vi "GC EX Vacuum - Step 1.vi"(7 "Step":i32, 8 "error in":errorcluster, 9 "Test Results In":T8, 10 "Gas":T1, 11 "GC Configuration":T2) -> (0 "error out":errorcluster, 1 "Test Results Out":T8, 2 "Gas Out":T1 caption="Gas", 3 "GC Configuration Out":T2)   [LabVIEW 2015]
uses:
  Controls/Test Information.ctl
  Controls/Vacuum Test.ctl
  Controls/Test Timing.ctl
  Controls/Vaccum Thresholds.ctl
  Controls/Helium Test.ctl
  Controls/Helium Thresholds.ctl
  CAN Communication/Gas/Typedefs/Session Handle.ctl
  CAN Communication/Gas/Gas.lvclass
  Controls/Test Results.ctl
  Controls/Step Result.ctl
  SubVIs/Timing/Timing.lvlib
panel:
  out "NI-DAQ Pressure":dbl
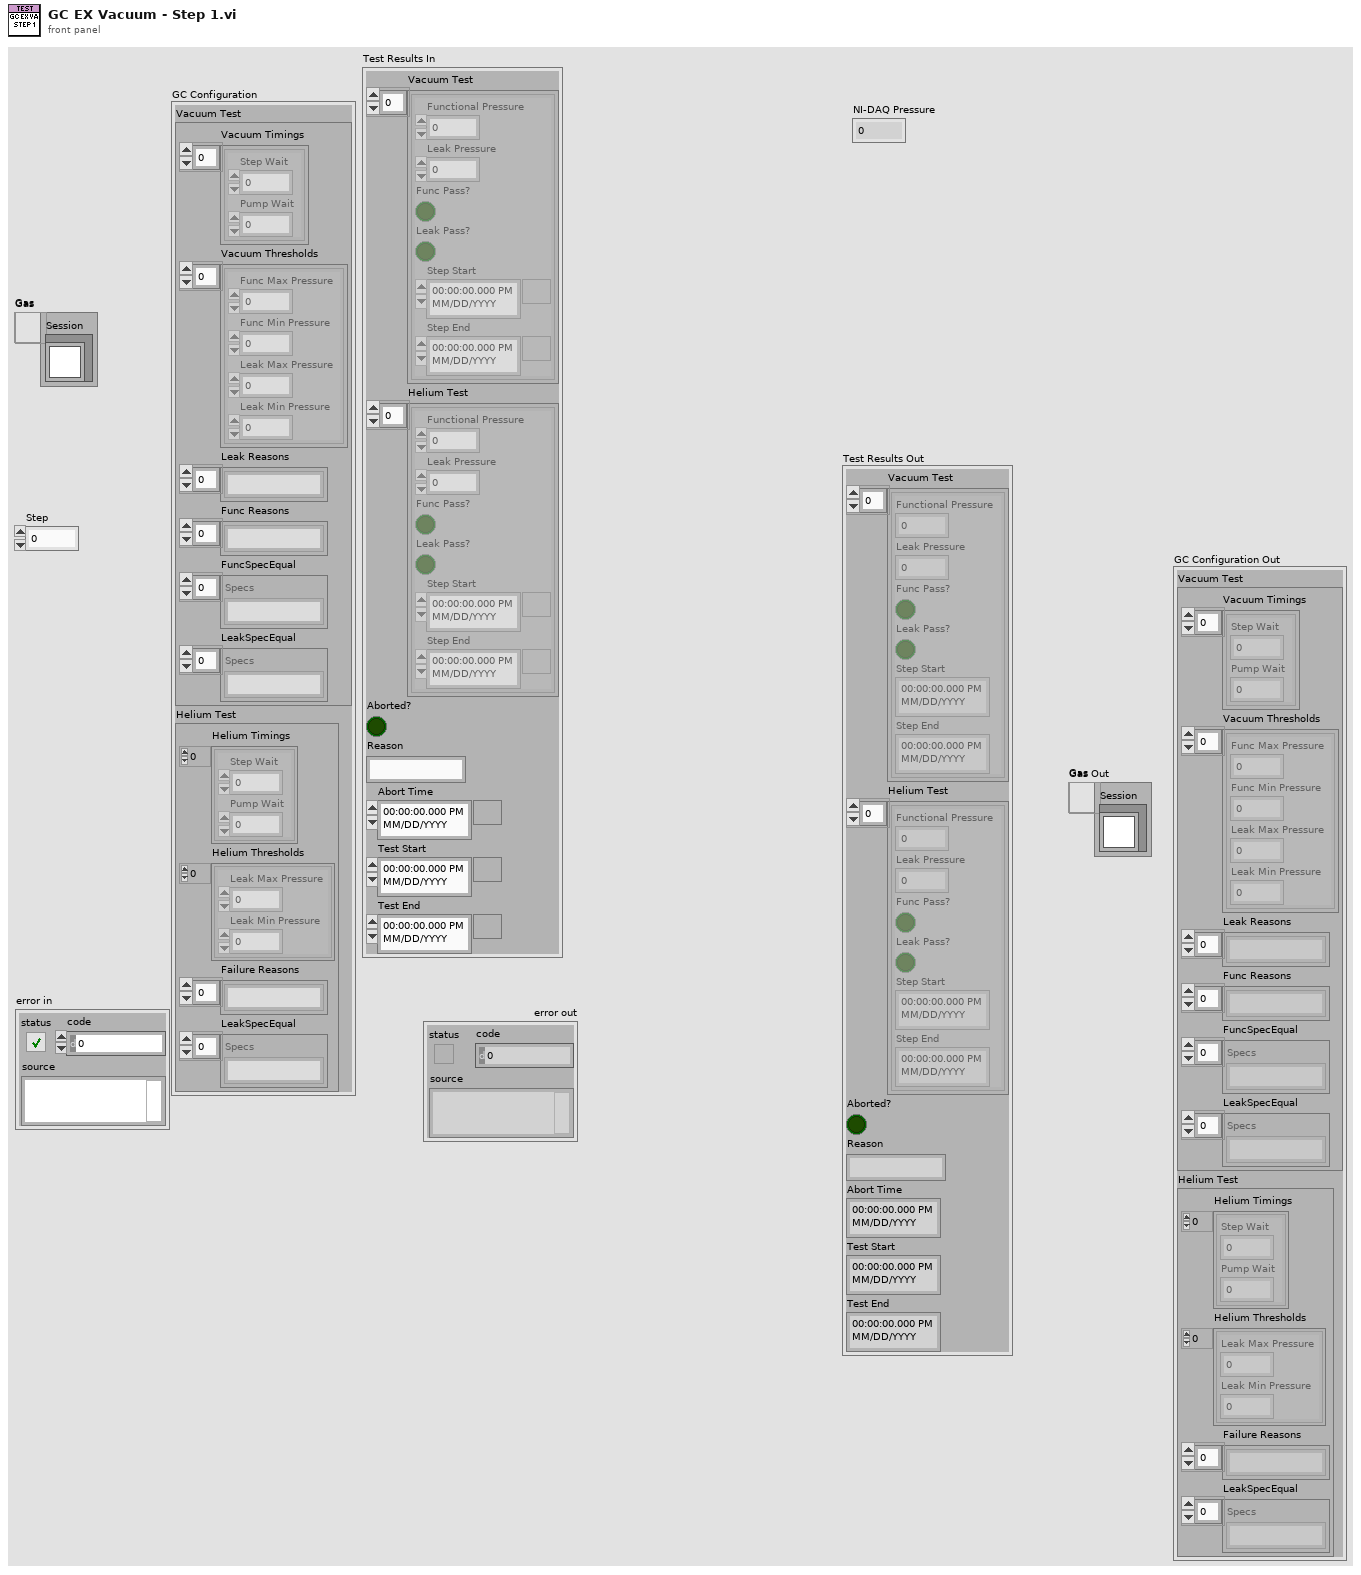
[diagram p1: front panel]
types:
  T1 = typedef "Gas.lvclass/Session Handle.ctl" = refnum<data-value>
  T2 = typedef "Test Information.ctl" = cluster{"Vacuum Test":T3, "Helium Test":T6}
  T3 = typedef "Vacuum Test.ctl" = cluster{"Vacuum Timings":T4[], "Vacuum Thresholds":T5[], "Leak Reasons":string[], "Func Reasons":string[], "FuncSpecEqual":string[], "LeakSpecEqual":string[]}
  T4 = typedef "Test Timing.ctl" = cluster{"Step Wait":dbl, "Pump Wait":dbl}
  T5 = typedef "Vaccum Thresholds.ctl" = cluster{"Func Max Pressure":dbl, "Func Min Pressure":dbl, "Leak Max Pressure":dbl, "Leak Min Pressure":dbl}
  T6 = typedef "Helium Test.ctl" = cluster{"Helium Timings":T4[], "Helium Thresholds":T7[], "Failure Reasons":string[], "LeakSpecEqual":string[]}
  T7 = typedef "Helium Thresholds.ctl" = cluster{"Leak Max Pressure":dbl, "Leak Min Pressure":dbl}
  T8 = typedef "Test Results.ctl" = cluster{"Vacuum Test":T9[], "Helium Test":T9[], "Aborted?":bool, "Reason":string, "Abort Time":timestamp, "Test Start":timestamp, "Test End":timestamp}
  T9 = typedef "Step Result.ctl" = cluster{"Functional Pressure":dbl, "Leak Pressure":dbl, "Func Pass?":bool, "Leak Pass?":bool, "Step Start":timestamp, "Step End":timestamp}
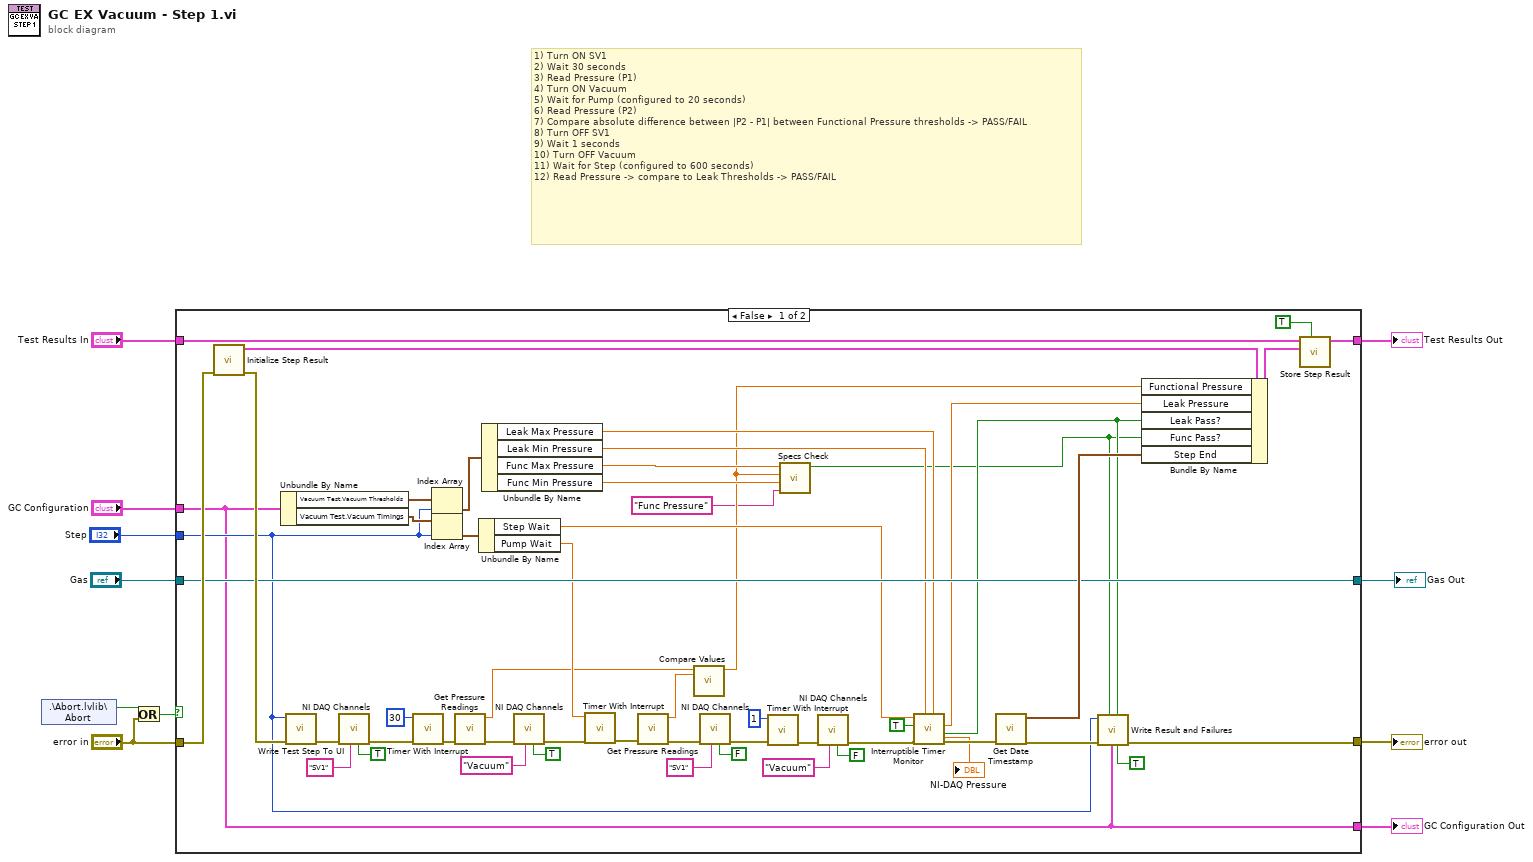
[diagram p0: block diagram]
diagram:
  # "1) Turn ON SV1\n2) Wait 30 seconds\n3) Read Pressure (P1)\n4) Turn ON Vacuum\n5) Wait for Pump (configured to 20 seconds)\n6) Read Pressure (P2)\n7) Compare absolute difference between |P2 - P1| between Functional Pressure thresholds -> PASS/FAIL\n8) Turn OFF SV1\n9) Wait 1 seconds\n10) Turn OFF Vacuum\n11) Wait for Step (configured to 600 seconds)\n12) Read Pressure -> compare to Leak Thresholds -> PASS/FAIL"
  n1 = shared-variable ".\\Abort.lvlib\\Abort"() -> (w10:bool)  [unwired: 1 in, 1 out]
  n2 = Or(x=w10, y="error in") -> (x .or. y?=w9:bool)
  n3 = case shown="False" w9 {
    tunnel: "error in" -> [w65 w68]
    tunnel: "Test Results In" -> [w62 w69]
    tunnel: [w63 w69] -> w7
    tunnel: [w45 w68] -> w6
    tunnel: "GC Configuration" -> [w43 w67]
    tunnel: "Step" -> [w44 _]
    tunnel: [w43 w67] -> w3
    tunnel: [w55 w66] -> w1
    tunnel: "Gas" -> [w55 w66]
    frame False {
      n4 = call "Initialize Step Result.vi"("error in (no error)"=w65) -> ("error out"=w64:errorcluster, "New Step Result"=w61:T9)  [unwired: 8 in, 1 out]
      n5 = Unbundle By Name(w43) -> ("Vacuum Test.Vacuum Thresholds"=w58:T5[], "Vacuum Test.Vacuum Timings"=w57:T4[])
      n6 = call "Write Test Step To UI.vi"("error in (no error)"=w64, "Step"=w44) -> ("error out"=w40:errorcluster)  [unwired: 9 in]
      n7 = call "NI DAQ Channels.vi"("Control"=TRUE ("State"), "Channel"="SV1", "error in (no error)"=w40) -> ("error out"=w39:errorcluster)  [unwired: 7 in, 1 out]
      n8 = call "Timer With Interrupt.vi"("error in (no error)"=w39, "Wait (s)"=30) -> ("error out"=w53:errorcluster)  [unwired: 7 in, 2 out]
      n9 = Index Array(array=w58, index=w44) -> (element=w51:T5)
      n10 = Index Array(array=w57, index=w44) -> (element=w56:T4)
      n11 = call "Get Pressure Readings.vi"("error in (no error)"=w53) -> ("error out"=w37:errorcluster, "NI-DAQ Pressure"=w48:dbl)  [unwired: 6 in, 3 out]
      n12 = Unbundle By Name(w56) -> ("Step Wait"=w27:dbl, "Pump Wait"=w52:dbl)
      n13 = Unbundle By Name(w51) -> ("Leak Max Pressure"=w24:dbl, "Leak Min Pressure"=w25:dbl, "Func Max Pressure"=w16:dbl, "Func Min Pressure"=w15:dbl)
      n14 = call "NI DAQ Channels.vi"("Control"=TRUE ("State"), "Channel"="Vacuum", "error in (no error)"=w37) -> ("error out"=w36:errorcluster)  [unwired: 7 in, 1 out]
      n15 = call "Timer With Interrupt.vi"("error in (no error)"=w36, "Wait (s)"=w52) -> ("error out"=w50:errorcluster)  [unwired: 7 in, 2 out]
      n16 = call "Get Pressure Readings.vi"("error in (no error)"=w50) -> ("error out"=w34:errorcluster, "NI-DAQ Pressure"=w49:dbl)  [unwired: 6 in, 3 out]
      n17 = call "Compare Values.vi"("P2"=w49, "P1"=w48) -> ("Abs Diff"=w14:dbl)  [unwired: 9 in]
      n18 = call "NI DAQ Channels.vi"("Control"=FALSE ("State"), "Channel"="SV1", "error in (no error)"=w34) -> ("error out"=w33:errorcluster)  [unwired: 7 in, 1 out]
      n19 = call "Timer With Interrupt.vi"("error in (no error)"=w33, "Wait (s)"=1) -> ("error out"=w31:errorcluster)  [unwired: 7 in, 2 out]
      n20 = call "Specs Check.vi"("parameter"="Func Pressure", "lower limit"=w15, "x"=w14, "upper limit"=w16) -> ("In Range?"=w13:bool)  [unwired: 6 in, 1 out]
      n21 = call "NI DAQ Channels.vi"("Control"=FALSE ("State"), "Channel"="Vacuum", "error in (no error)"=w31) -> ("error out"=w29:errorcluster)  [unwired: 7 in, 1 out]
      n22 = call "Interruptible Timer Monitor.vi"("Max"=w24, "Min"=w25, "error in (no error)"=w29, "Update UI?"=TRUE, "Wait (s)"=w27) -> ("error out"=w28:errorcluster, "In Range?"=w22:bool, "Leak Rate"=w23:dbl, "NI-DAQ Pressure"=→"NI-DAQ Pressure":dbl)  [unwired: 2 in, 1 out]
      n23 = call "Get Date Timestamp.vi"("error in (no error)"=w28) -> ("error out"=w46:errorcluster, "current time"=w59:timestamp)  [unwired: 9 in]
      n24 = call "Write Result and Failures.vi"("Vacuum?"=TRUE, "Leak"=w22, "GC Configuration"=w43, "Func"=w13, "error in (no error)"=w46, "Step"=w44) -> ("error out"=w45:errorcluster)  [unwired: 5 in]
      n25 = Bundle By Name(cluster=w61, "Functional Pressure"=w14, "Leak Pressure"=w23, "Leak Pass?"=w22, "Func Pass?"=w13, "Step End"=w59) -> (w60:T9)
      n26 = call "Store Step Result.vi"("Vacuum?"=TRUE, "Step Result"=w60, "Test Results In"=w62) -> ("Test Results Out"=w63:T8)  [unwired: 8 in]
    }
    frame True {
    }
  }
  "error out" <- w6
  "Test Results Out" <- w7
  "GC Configuration Out" <- w3
  "Gas Out" <- w1
